vi "Clean.vi"   [LabVIEW 2017, in "Scripts.lvlib"]
doc: "Deletes the \"target\" and \"builds\" folders in the project root."
uses:
  Scripts.lvlib
panel:
  # "Overview: Deletes the artifacts for building and packaging\nRequirements: LabVIEW\nInstructions: Run this VI.\n\nDeletes the \"builds\" and \"target\" folders if they exist in the project root. Use with caution."
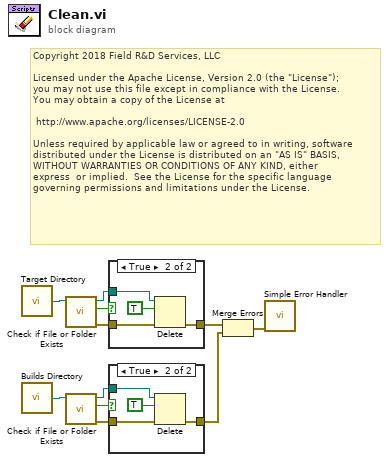
[diagram p0: block diagram]
diagram:
  # "Copyright 2018 Field R&D Services, LLC\n\nLicensed under the Apache License, Version 2.0 (the \"License\");\nyou may not use this file except in compliance with the License.\nYou may obtain a copy of the License at\n\n\thttp://www.apache.org/licenses/LICENSE-2.0\n\nUnless required by applicable law or agreed to in writing, software\ndistributed under the License is distributed on an \"AS IS\" BASIS,\nWITHOUT WARRANTIES OR CONDITIONS OF ANY KIND, either \nexpress  or implied.  See the License for the specific language \ngoverning permissions and limitations under the License."
  n1 = call "Target Directory.vi"() -> ("Target Directory"=w1:path)
  n2 = call "Builds Directory.vi"() -> ("Builds Directory"=w8:path)
  n3 = call <vilib>:"Check if File or Folder Exists.vi"("path"=w1) -> ("error out"=w10:errorcluster, "file or folder exists?"=w11:bool, "dup path"=w9:path)  [unwired: 8 in]
  n4 = call <vilib>:"Check if File or Folder Exists.vi"("path"=w8) -> ("error out"=w5:errorcluster, "file or folder exists?"=w7:bool, "dup path"=w6:path)  [unwired: 8 in]
  n5 = case shown="True" w11 {
    tunnel: w10 -> [w12 w14]
    tunnel: w9 -> [_ w16]
    tunnel: [w12 w13] -> w4
    frame False {
    }
    frame True {
      n6 = Delete(path (use dialog)=w16, entire hierarchy (F)=TRUE, error in=w14) -> (error out=w13:errorcluster)  [unwired: 2 in, 2 out]
    }
  }
  n7 = case shown="True" w7 {
    tunnel: w5 -> [w17 w19]
    tunnel: w6 -> [_ w21]
    tunnel: [w17 w18] -> w3
    frame False {
    }
    frame True {
      n8 = Delete(path (use dialog)=w21, entire hierarchy (F)=TRUE, error in=w19) -> (error out=w18:errorcluster)  [unwired: 2 in, 2 out]
    }
  }
  n9 = Merge Errors(w4, w3) -> (w2:errorcluster)
  n10 = call <vilib>:"Simple Error Handler.vi"("error in (no error)"=w2) -> ()  [unwired: 4 in, 5 out]
